vi "Reorganize&ScaleMeasurements.vi"(7 "MeasurementType":string, 8 "Error In":errorcluster, 10 "Register Values":u16[](array[numeric]), 11 "Measurement TextRing":u16) -> (0 "Error Out":errorcluster, 1 "Numerical Information":bool, 2 "String":string, 3 "output waveform":waveform(dbl))   [LabVIEW 2018, in "SensorPlugins.lvlib" / "SiemensDigitalEnergyMeter.lvclass"]
doc: "This VI takes the raw measurements from the Siemens Digital Energy Meter. It scales the measurements accordingly and separates the measurements between numerical and status measurements."
uses:
  SiemensDigitalEnergyMeter.lvclass
  <vilib>/Utility/error.llb/Error Cluster From Error Code.vi
  <vilib>/ErrorRing/Error Ring.xnode
panel:
  out "replaced":bool
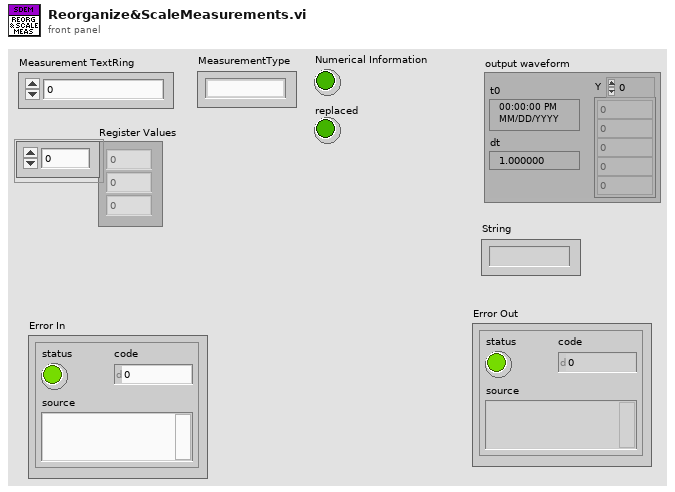
[diagram p1: front panel]
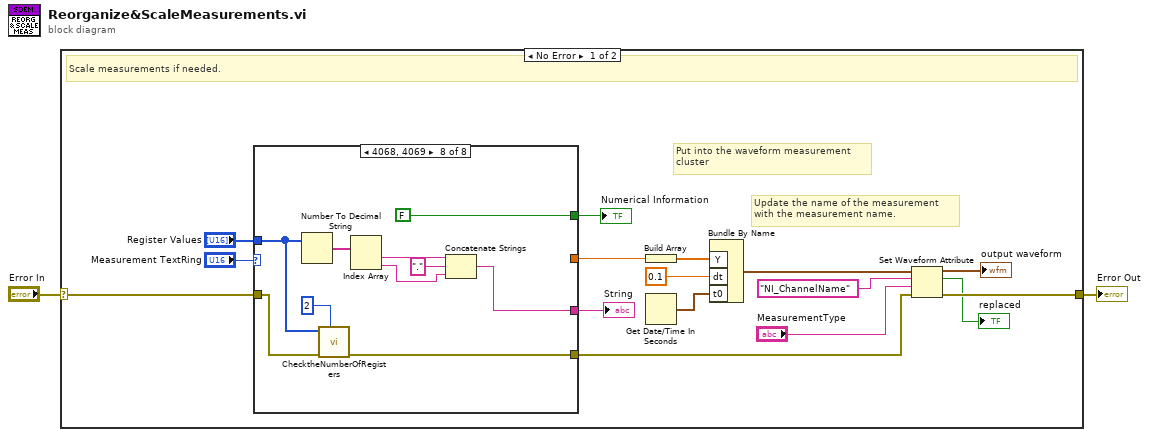
[diagram p0: block diagram]
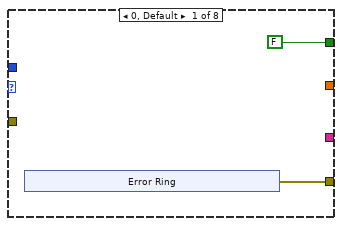
[diagram p2: hidden frame]
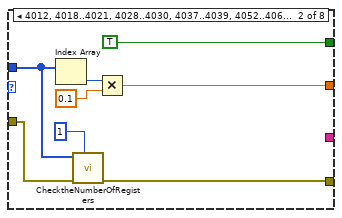
[diagram p3: hidden frame]
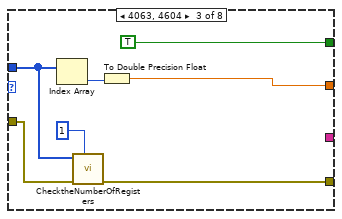
[diagram p4: hidden frame]
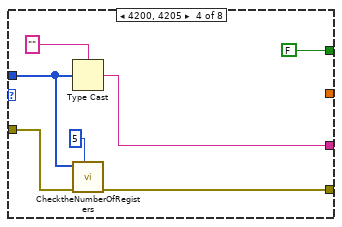
[diagram p5: hidden frame]
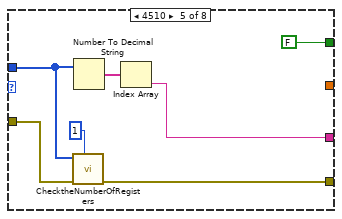
[diagram p6: hidden frame]
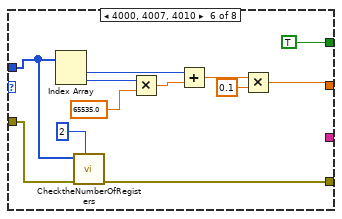
[diagram p7: hidden frame]
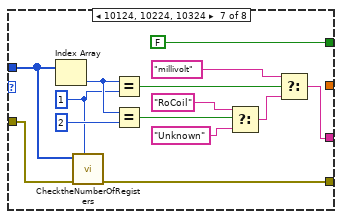
[diagram p8: hidden frame]
diagram:
  n1 = case shown="No Error" "Error In" {
    selector: "Error In" -> [w4 w91]
    tunnel: [w8 w91] -> w2
    frame No Error {
      # "Update the name of the measurement \nwith the measurement name."
      # "Put into the waveform measurement\ncluster"
      # "Scale measurements if needed."
      n2 = case shown="4068, 4069" "Measurement TextRing" {
        tunnel: "Register Values" -> [_ w26 w34 w44 w49 w55 w69 w81]
        tunnel: [_ w31 w39 _ _ w59 _ _] -> w11
        tunnel: [_ _ _ w45 w48 _ w67 w85] -> w17
        tunnel: [FALSE ("Numerical Information") TRUE ("Numerical Information") TRUE ("Numerical Information") FALSE ("Numerical Information") FALSE ("Numerical Information") TRUE ("Numerical Information") FALSE ("Numerical Information") FALSE ("Numerical Information")] -> w15
        tunnel: w4 -> [_ w28 w36 w42 w52 w58 w71 w83]
        tunnel: [w19 w27 w35 w43 w53 w56 w70 w82] -> w3
        frame 0, Default {
          n3 = xnode "Error Ring"() -> ("error out"=w19:errorcluster)
        }
        frame 4012, 4018..4021, 4028..4030, 4037..4039, 4052..4060 {
          n4 = Index Array(array=w26) -> (element=w33:u16)  [unwired: 1 in]
          n5 = call "ChecktheNumberOfRegisters.vi"("Number of Registers"=1 ("x"), "error in (no error)"=w28, "Register Values"=w26) -> ("error out"=w27:errorcluster)  [unwired: 8 in]
          n6 = Multiply(x=w33, y=0.1) -> (x*y=w31:dbl)
        }
        frame 4063, 4604 {
          n7 = Index Array(array=w34) -> (element=w40:u16)  [unwired: 1 in]
          n8 = call "ChecktheNumberOfRegisters.vi"("Number of Registers"=1 ("x"), "error in (no error)"=w36, "Register Values"=w34) -> ("error out"=w35:errorcluster)  [unwired: 8 in]
          n9 = To Double Precision Float(number=w40) -> (double precision float=w39:dbl)
        }
        frame 4200, 4205 {
          n10 = Type Cast(type="", x=w44) -> (*(type *) &x=w45:string)
          n11 = call "ChecktheNumberOfRegisters.vi"("Number of Registers"=5 ("x"), "error in (no error)"=w42, "Register Values"=w44) -> ("error out"=w43:errorcluster)  [unwired: 8 in]
        }
        frame 4510 {
          n12 = call "ChecktheNumberOfRegisters.vi"("Number of Registers"=1 ("x"), "error in (no error)"=w52, "Register Values"=w49) -> ("error out"=w53:errorcluster)  [unwired: 8 in]
          n13 = Number To Decimal String(number=w49) -> (decimal integer string=w50:string[])  [unwired: 1 in]
          n14 = Index Array(array=w50) -> (element=w48:string)  [unwired: 1 in]
        }
        frame 4000, 4007, 4010 {
          n15 = Index Array(array=w55) -> (element #1=w62:u16, element #2=w65:u16)  [unwired: 2 in]
          n16 = call "ChecktheNumberOfRegisters.vi"("Number of Registers"=2 ("x"), "error in (no error)"=w58, "Register Values"=w55) -> ("error out"=w56:errorcluster)  [unwired: 8 in]
          n17 = Multiply(x=w65, y=65535.0 ("x")) -> (x*y=w63:dbl)
          n18 = Add(x=w62, y=w63) -> (x+y=w61:dbl)
          n19 = Multiply(x=w61, y=0.1) -> (x*y=w59:dbl)
        }
        frame 10124, 10224, 10324 {
          w68 = u16 1 ("y")
          n20 = Index Array(array=w69) -> (element=w75:u16)  [unwired: 1 in]
          n21 = call "ChecktheNumberOfRegisters.vi"("Number of Registers"=w68, "error in (no error)"=w71, "Register Values"=w69) -> ("error out"=w70:errorcluster)  [unwired: 8 in]
          n22 = Equal?(x=w75, y=w68) -> (x = y?=w77:bool)
          n23 = Equal?(x=w75, y=u16 2) -> (x = y?=w74:bool)
          n24 = Select(t="RoCoil" ("f"), s=w74, f="Unknown") -> (s? t:f=w79:string)
          n25 = Select(t="millivolt" ("String"), s=w77, f=w79) -> (s? t:f=w67:string)
        }
        frame 4068, 4069 {
          n26 = Number To Decimal String(number=w81) -> (decimal integer string=w89:string[])  [unwired: 1 in]
          n27 = call "ChecktheNumberOfRegisters.vi"("Number of Registers"=2 ("x"), "error in (no error)"=w83, "Register Values"=w81) -> ("error out"=w82:errorcluster)  [unwired: 8 in]
          n28 = Index Array(array=w89) -> (element #1=w88:string, element #2=w86:string)  [unwired: 2 in]
          n29 = Concatenate Strings(w88, "." ("string"), w86) -> (w85:string)
        }
      }
      "String" <- w17
      "Numerical Information" <- w15
      n30 = Build Array(w11) -> (w14:dbl[])
      n31 = Get Date/Time In Seconds() -> (seconds since 1Jan1904=w13:timestamp)
      n32 = Bundle By Name("Y"=w14, "dt"=0.1, "t0"=w13) -> (w10:waveform(dbl))  [unwired: 1 in]
      n33 = Set Waveform Attribute(4:w3, 5:"MeasurementType", 6:"NI_ChannelName" ("name"), 7:w10) -> (0:w8:errorcluster, 2:→"replaced":bool, 3:→"output waveform":waveform(dbl))
    }
    frame Error {
    }
  }
  "Error Out" <- w2
